vi "Start Calibration.vi"(8 "error in (no error)":errorcluster, 10 "Calibration Type (0:Open)":u32(ring) items=["Open", "Short", "Zero Continuity", "Zero Resistance", "Standard"], 11 "VISA resource name":refnum<visa-resource-name>) -> (0 "error out":errorcluster, 3 "VISA resource name out":refnum<visa-resource-name>)   [LabVIEW 2010, in "Agilent 4194.lvlib"]
doc: "This function starts particular calibration."
uses:
  <instrlib>/Agilent 4194/Agilent 4194.lvlib
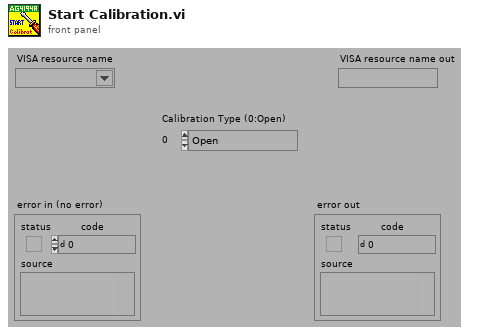
[diagram p1: front panel]
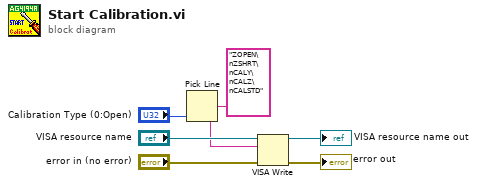
[diagram p0: block diagram]
diagram:
  n1 = Pick Line(multi-line string="ZOPEN\nZSHRT\nCALY\nCALZ\nCALSTD", line index="Calibration Type (0:Open)") -> (output string=w1:string)  [unwired: 1 in]
  n2 = VISA Write(VISA resource name="VISA resource name", write buffer=w1, error in (no error)="error in (no error)") -> (VISA resource name out=→"VISA resource name out":refnum<visa-resource-name>, error out=→"error out":errorcluster)  [unwired: 1 out]
